vi "ma_Tone estimation.vi"   [LabVIEW 2020, in "NI_MAPro.lvlib"]
uses:
  NI_MAPro.lvlib
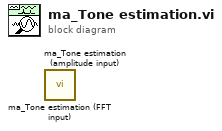
[diagram p0: block diagram]
diagram:
  n1 = call "ma_Tone estimation (FFT input).vi"() -> ()  [unwired: 2 in, 1 out]
  n2 = call "ma_Tone estimation (amplitude input).vi"() -> ()  [unwired: 2 in, 1 out]
